vi "Stepper Command.vi"(8 "Microstep Coil Activation":dbl[](array[numeric]), 9 "Microstep Enable":bool, 10 "Stepper Coil Activation":bool[](array[boolean]), 11 "IO Cluster IN":T1) -> (0 "Error Out":errorcluster, 3 "IO Cluster OUT":T1)   [LabVIEW 2019]
uses:
  Actuators IO Cluster.ctl
  <vilib>/Utility/error.llb/Error Cluster From Error Code.vi
  <vilib>/rvi/errors/niLvFpgaAdjustHostInterfaceError.vi
  <vilib>/rvi/interface/nirviReadWriteControl/nirviReadWriteControl.xnode
  NiFpgaLv.dll
  <vilib>/rvi/interface/Simulation/niFpgaSimulationCallBeginRW.vi
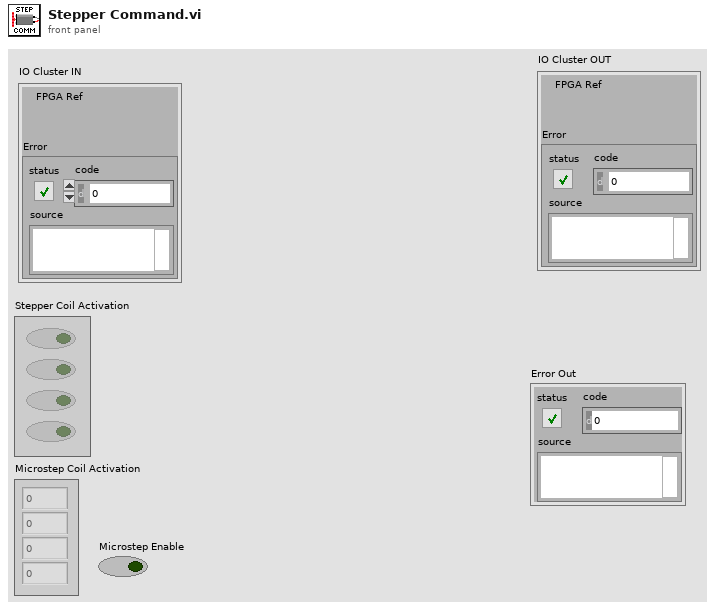
[diagram p1: front panel]
types:
  T1 = typedef "Actuators IO Cluster.ctl" = cluster{"Error":errorcluster, "FPGA Ref":refnum<k20>}
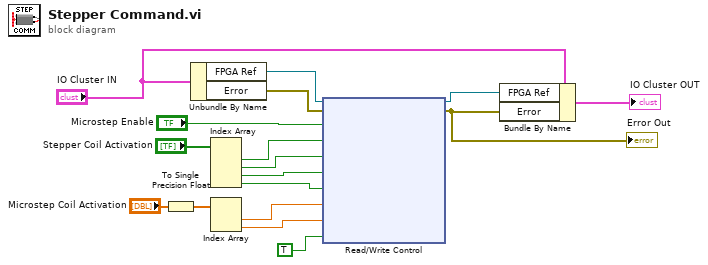
[diagram p0: block diagram]
diagram:
  n1 = To Single Precision Float(number="Microstep Coil Activation") -> (single precision float=w5:sgl[])
  n2 = Unbundle By Name("IO Cluster IN") -> ("FPGA Ref"=w3:refnum<k20>, "Error"=w2:errorcluster)
  n3 = Index Array(array="Stepper Coil Activation") -> (element #1=w14:bool, element #2=w13:bool, element #3=w12:bool, element #4=w11:bool)  [unwired: 4 in]
  n4 = Index Array(array=w5) -> (element #1=w7:sgl, element #2=w4:sgl)  [unwired: 2 in]
  n5 = xnode "Read/Write Control"("FPGA VI引用输入"=w3, "错误输入"=w2, "Microstep Enable"="Microstep Enable", "Stepper Control 1"=w14, "Stepper Control 2"=w13, "Stepper Control 3"=w12, "Stepper Control 4"=w11, "Microstep AC"=w7, "Microstep BD"=w4, "LED Stepper"=TRUE ("LED DC Motor")) -> ("FPGA VI引用输出"=w10:refnum<k20>, "错误输出"=w16:errorcluster)
  "Error Out" <- w16
  n6 = Bundle By Name(cluster="IO Cluster IN", "FPGA Ref"=w10, "Error"=w16) -> (→"IO Cluster OUT":T1)
